vi "Programmed Temperature for Step N.vi"(11 "Step #":i32) -> (1 "New Temperature  Message":string, 3 "Desired Temperature":dbl)   [LabVIEW 2025, in "Programmatic Controller.lvclass"]
doc: "Given the step number, return the desired temperature to be maintained in that step in both numeric and string form."
uses:
  Programmatic Controller.lvclass
panel:
  in  "New Desired Temperature Message":string="New desired temperature: %d"
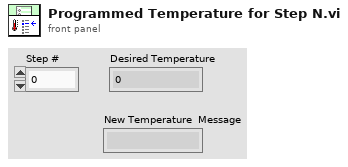
[diagram p1: front panel]
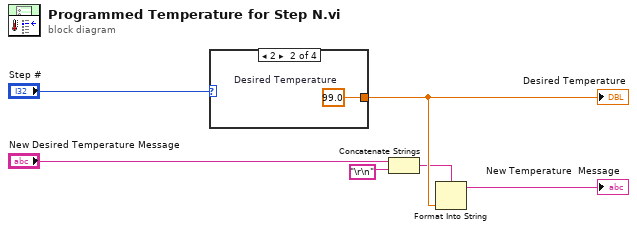
[diagram p0: block diagram]
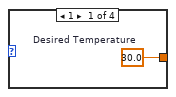
[diagram p2: hidden frame]
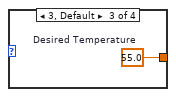
[diagram p3: hidden frame]
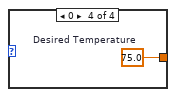
[diagram p4: hidden frame]
diagram:
  n1 = case shown="2" "Step #" {
    tunnel: [w7 w8 w9 w10] -> w5
    frame 1 {
      w7 = 30.0  # Desired Temperature
    }
    frame 2 {
      w8 = 99.0  # Desired Temperature
    }
    frame 3, Default {
      w9 = 55.0  # Desired Temperature
    }
    frame 0 {
      w10 = 75.0  # Desired Temperature
    }
  }
  "Desired Temperature" <- w5
  n2 = Concatenate Strings("New Desired Temperature Message", "\r\n") -> (w2:string)
  n3 = Format Into String(format string=w2, w5) -> (resulting string=→"New Temperature  Message":string)  [unwired: 2 in, 1 out]
